vi "Boolean Output Item.vi"(8 "error in (no error)":errorcluster, 9 "Project In":refnum<class "Project.lvclass">, 11 "Output":T2) -> (0 "error out":errorcluster)   [LabVIEW 2015, in "OutputUI.lvclass"]
uses:
  OutputUI.lvclass
  Step/STEP_OUTPUT.ctl
  Step/OUTPUT_DATA_TYPE.ctl
  OUTPUT_CHECK_TYPE.ctl
  Step/OUTPUT_VALUE_TYPE.ctl
  Project.lvclass
  SerializableObject/CONFIGURE_UI_STATE.ctl
  Editor/Editor.lvclass
  Step.lvclass
panel:
  in  "Limit Value Type":T1
  in  "Variable Name":string(combo) caption="Variable Name 1"
  in  "Boolean Limit":bool
  in  "Check":u16(ring)
  out "Type Image":picture
  in  "Output":string
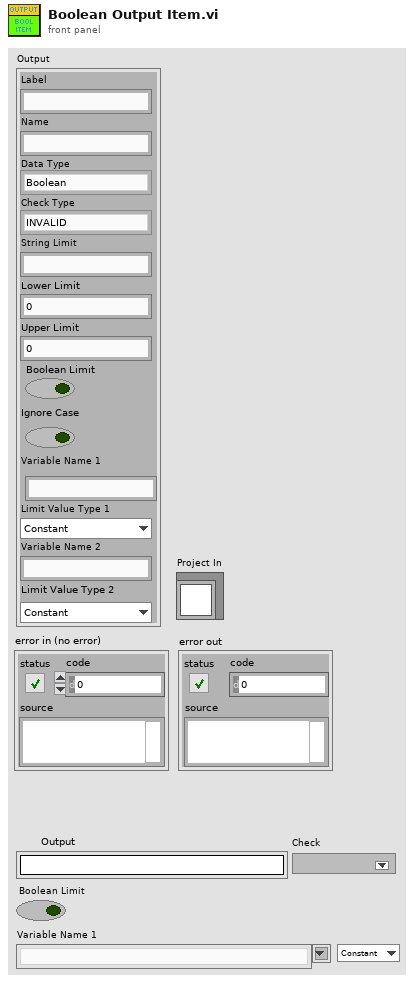
[diagram p1: front panel]
types:
  T1 = typedef "Step.lvclass/OUTPUT_VALUE_TYPE.ctl" = enum16{"Constant", "Variable"}
  T2 = typedef "Step.lvclass/STEP_OUTPUT.ctl" = cluster{"Label":string, "Name":string, "Data Type":T3, "Check Type":T4, "String Limit":string, "Lower Limit":dbl, "Upper Limit":dbl, "Boolean Limit":bool, "Ignore Case":bool, "Variable Name 1":string, "Limit Value Type 1":T1, "Variable Name 2":string, "Limit Value Type 2":T1}
  T3 = typedef "Step.lvclass/OUTPUT_DATA_TYPE.ctl" = enum16{"Boolean", "String", "Numeric", "Other"}
  T4 = typedef "Step.lvclass/OUTPUT_CHECK_TYPE.ctl" = enum16{"INVALID", "DO_NOT_CHECK", "RECORD", "VARIABLE", "EQUAL", "NOT_EQUAL", "STR_CONTAINS", "STR_START_WITH", "STR_END_WITH", "STR_REGEX_MATCH", "NUM_GT", "NUM_LT", "NUM_GE", "NUM_LE", "NUM_RANGE", "NUM_RANGE_BDY"}
  T5 = cluster{"Type Image":refnum<vi>, "Output":refnum<vi>, "Check":refnum<vi>, "Boolean Limit":refnum<vi>, "Variable Name":refnum<vi>, "Limit Value Type":refnum<vi>}
  T6 = typedef "Editor.lvclass/CONFIGURE_UI_STATE.ctl" = enum16{"UI_LOOP", "INIT", "END", "CHANGE_PANEL"}
  T7 = typedef "LVRectTypeDef.ctl" = cluster{"Left":i16, "Top":i16, "Right":i16, "Bottom":i16}
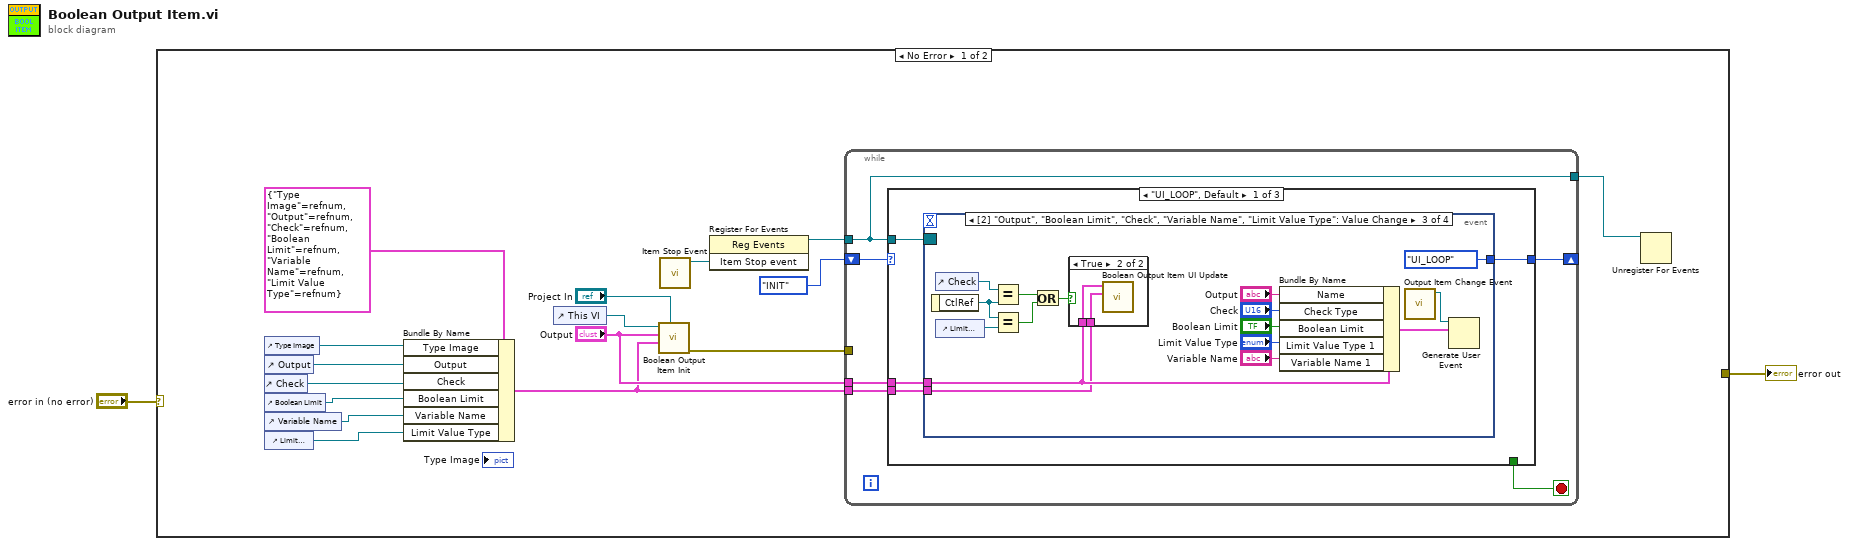
[diagram p0: block diagram]
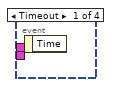
[diagram p2: hidden frame]
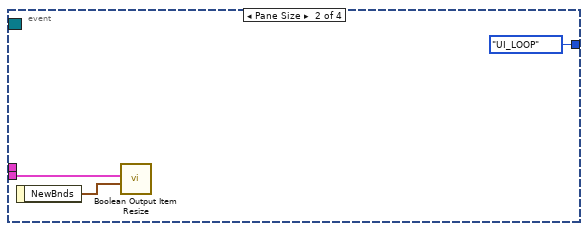
[diagram p3: hidden frame]
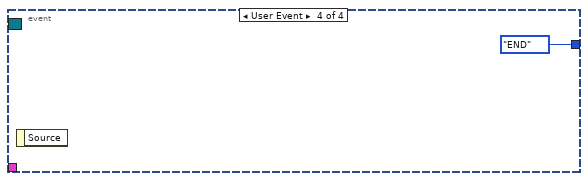
[diagram p5: hidden frame]
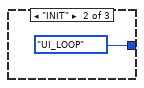
[diagram p6: hidden frame]
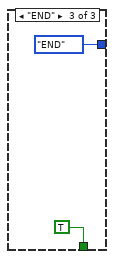
[diagram p7: hidden frame]
diagram:
  n1 = case shown="No Error" "error in (no error)" {
    selector: "error in (no error)" -> [_ w54]
    tunnel: [_ w54] -> w1
    frame No Error {
      n2 = control-ref of="Type Image"() -> (w11:refnum<vi>)
      n3 = control-ref of="Output"() -> (w8:refnum<vi>)
      n4 = control-ref of="Check"() -> (w9:refnum<vi>)
      n5 = control-ref of="Boolean Limit"() -> (w6:refnum<vi>)
      n6 = control-ref of="Variable Name"() -> (w5:refnum<vi>)
      n7 = control-ref of="Limit Value Type 1"() -> (w4:refnum<vi>)
      n8 = Bundle By Name(cluster=T5 {"Type Image"=refnum, "Output"=refnum, "Check"=refnum, "Boolean Limit"=refnum, "Variable Name"=refnum, "Limit Value Type"=refnum} ("UI Elements"), "Type Image"=w11, "Output"=w8, "Check"=w9, "Boolean Limit"=w6, "Variable Name"=w5, "Limit Value Type"=w4) -> (w3:T5)
      n9 = control-ref of="This VI"() -> (w14:refnum<vi>)
      n10 = call "Boolean Output Item Init.vi"("Project In"="Project In", "Bool UI Elements"=w3, "Output"="Output", "VI in"=w14) -> ("error out"=w13:errorcluster)  [unwired: 7 in]
      n11 = call "Item Stop Event.vi"() -> ("Item Stop event"=w17:refnum<user-event>)  [unwired: 11 in]
      n12 = register-events(w17) -> (reference out=w16:refnum<event-registration>)  [unwired: 2 in, 1 out]
      n13 = while {
        shift-right: [w23] -> _
        shift-left: CONFIGURE_UI_STATE."INIT" -> [w24]
        tunnel: w16 -> [w21]
        tunnel: [w21] -> w15
        tunnel: w13 -> [_]
        tunnel: "Output" -> [w20]
        tunnel: w3 -> [w19]
        stop <- w22 stop-if-true
        n14 = case shown="\"UI_LOOP\", Default" w24 {
          tunnel: [w28 CONFIGURE_UI_STATE."UI_LOOP" CONFIGURE_UI_STATE."END"] -> w23
          tunnel: [_ _ TRUE] -> w22
          tunnel: w21 -> [w27 _ _]
          tunnel: w20 -> [w26 _ _]
          tunnel: w19 -> [w25 _ _]
          frame "UI_LOOP", Default {
            n15 = event shown="[2] \"Output\", \"Boolean Limit\", \"Check\", \"Variable Name\", \"Limit Value Type\": Value Change" {
              selector: w27 -> [_ _ _ _]
              dyn-events: _ -> [_ _ _ _]
              timeout: _ -> [_ _ _ _]
              tunnel: [_ CONFIGURE_UI_STATE."UI_LOOP" CONFIGURE_UI_STATE."UI_LOOP" CONFIGURE_UI_STATE."END"] -> w28
              tunnel: w26 -> [_ _ w41 _]
              tunnel: w25 -> [_ w31 w40 _]
              event Timeout {
                n16 = event-data() -> ()  [unwired: 1 in, 1 out]
              }
              event Pane Size {
                n17 = event-data() -> ("NewBnds"=w30:T7)  [unwired: 1 in]
                n18 = call "Boolean Output Item Resize.vi"("NewBnds"=w30, "Bool UI Elements"=w31) -> ()  [unwired: 9 in, 1 out]
              }
              event "Output", "Boolean Limit", "Check", "Variable Name": Value Change {
                n19 = event-data() -> ("CtlRef"=w36:refnum<vi>)  [unwired: 1 in]
                n20 = control-ref of="Check"() -> (w42:refnum<vi>)
                n21 = control-ref of="Limit Value Type 1"() -> (w35:refnum<vi>)
                n22 = Equal?(x=w42, y=w36) -> (x = y?=w34:bool)
                n23 = Equal?(x=w36, y=w35) -> (x = y?=w33:bool)
                n24 = Or(x=w34, y=w33) -> (x .or. y?=w32:bool)
                n25 = case shown="True" w32 {
                  tunnel: w41 -> [_ w49]
                  tunnel: w40 -> [_ w48]
                  frame False {
                  }
                  frame True {
                    n26 = call "Boolean Output Item UI Update.vi"("Bool UI Elements"=w48, "Output"=w49) -> ()  [unwired: 9 in, 1 out]
                  }
                }
                n27 = Bundle By Name(cluster=w41, "Name"="Output", "Check Type"="Check", "Boolean Limit"="Boolean Limit", "Limit Value Type 1"="Limit Value Type", "Variable Name 1"="Variable Name") -> (w43:T2)
                n28 = call "Output Item Change Event.vi"() -> ("Output Value Change Event"=w44:refnum<user-event>)  [unwired: 11 in]
                n29 = Generate User Event(user event=w44, event data cluster=w43) -> ()  [unwired: 2 in, 2 out]
              }
              event User Event {
                n30 = event-data() -> ()  [unwired: 1 in, 1 out]
              }
            }
          }
          frame "INIT" {
          }
          frame "END" {
          }
        }
      }
      n31 = Unregister For Events(event registration refnum=w15) -> ()  [unwired: 1 in, 1 out]
    }
    frame Error {
    }
  }
  "error out" <- w1
